vi "HEWH Check C1 C2 Conditions.vi"(8 "Error In":errorcluster, 11 "Current Input":T1) -> (0 "Error Out":errorcluster, 3 "C1 or C2?":bool)   [LabVIEW 2019]
uses:
  Type Definitions/HEWH Special Condition Check.ctl
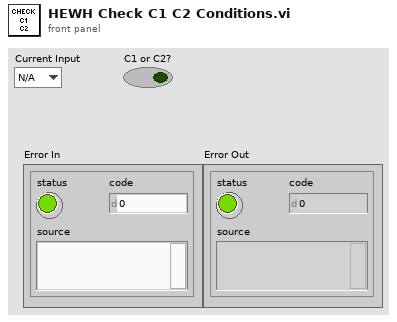
[diagram p1: front panel]
types:
  T1 = typedef "HEWH Special Condition Check.ctl" = enum16{"N/A", "C1", "C2", "Reset/Fail", "Skip Draw Sequence"}
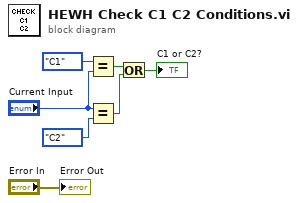
[diagram p0: block diagram]
diagram:
  n1 = Equal?(x=HEWH_Special_Condition_Check."C1" ("y"), y="Current Input") -> (x = y?=w4:bool)
  n2 = Equal?(x="Current Input", y=HEWH_Special_Condition_Check."C2") -> (x = y?=w5:bool)
  n3 = Or(x=w4, y=w5) -> (x .or. y?=→"C1 or C2?":bool)
  "Error Out" <- "Error In"
